vi "Tag Value.vi"() -> (3 "Tag Value":string)   [LabVIEW 2016]
doc: "Assign <B><tag></B> to the <B>Tag Value</B>"
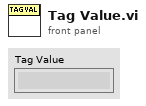
[diagram p1: front panel]
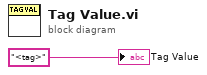
[diagram p0: block diagram]
diagram:
  "Tag Value" <- "<tag>"
